vi "Filter Zeroes.vi"(11 "Array in":u32[](array[numeric])) -> (3 "Array out":u32[](array[numeric]))   [LabVIEW 2013, in "Problem 18.lvlib"]
uses:
  Problem 18.lvlib
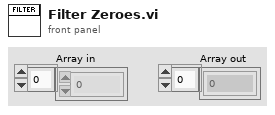
[diagram p1: front panel]
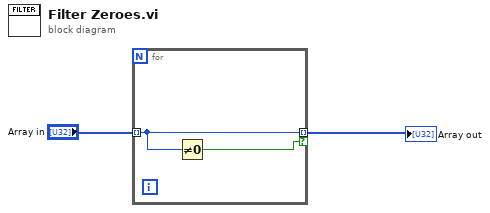
[diagram p0: block diagram]
diagram:
  n1 = for {
    tunnel: "Array in" -> [w4] mode=indexing
    tunnel: [w4] -> w1 mode=indexing if=w3
    n2 = Not Equal To 0?(x=w4) -> (x != 0?=w3:bool)
  }
  "Array out" <- w1
